vi "Read Config.vi"(8 "error in (no error)":errorcluster, 11 "ProjectLoader in":refnum<class "ProjectLoader.lvclass">) -> (0 "error out":errorcluster, 2 "Config":variant, 3 "ProjectLoader out":refnum<class "ProjectLoader.lvclass">)   [LabVIEW 2015, in "ProjectLoader.lvclass"]
uses:
  ProjectLoader.lvclass
  ProjectLoader.lvclass/ProjectLoader.ctl
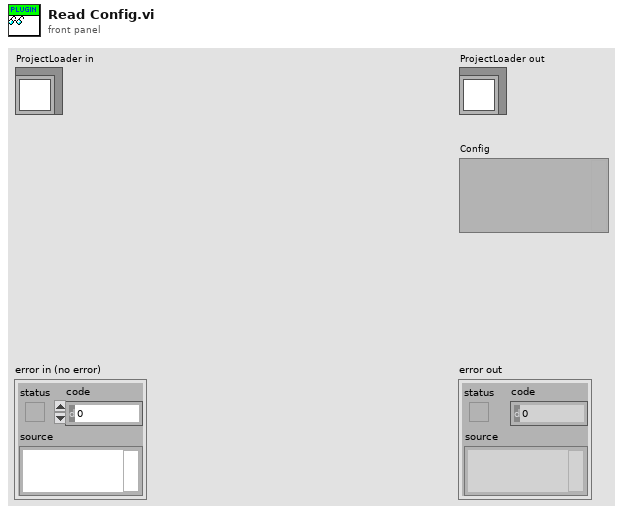
[diagram p1: front panel]
types:
  T1 = cluster{"Enable":bool, "Auto Load":bool, "Project File":path}
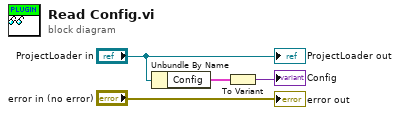
[diagram p0: block diagram]
diagram:
  n1 = Unbundle By Name("ProjectLoader in") -> ("Config"=w3:T1)
  n2 = To Variant(anything=w3) -> (Variant=→"Config":variant)
  "error out" <- "error in (no error)"
  "ProjectLoader out" <- "ProjectLoader in"
